vi "login_form.vi"() -> ()   [LabVIEW 2020]
uses:
  <vilib>/httpClient/MultipartData.ctl
  <vilib>/httpClient/LabVIEWHTTPClient.lvlib
panel:
  out "Round tab 2":i32
  in  "Tab Control":enum32{"login", "process"}(tab)
  in  "Cluster":T1
  in  "login":bool
  in  "data":T2[](array[typedef])
  out "Boolean 2":bool
  in  "Boolean":bool
  out "token":string
  out "Hello":string
  in  "stop":bool
  out "date now":string
  out "time":string
  out "body":string
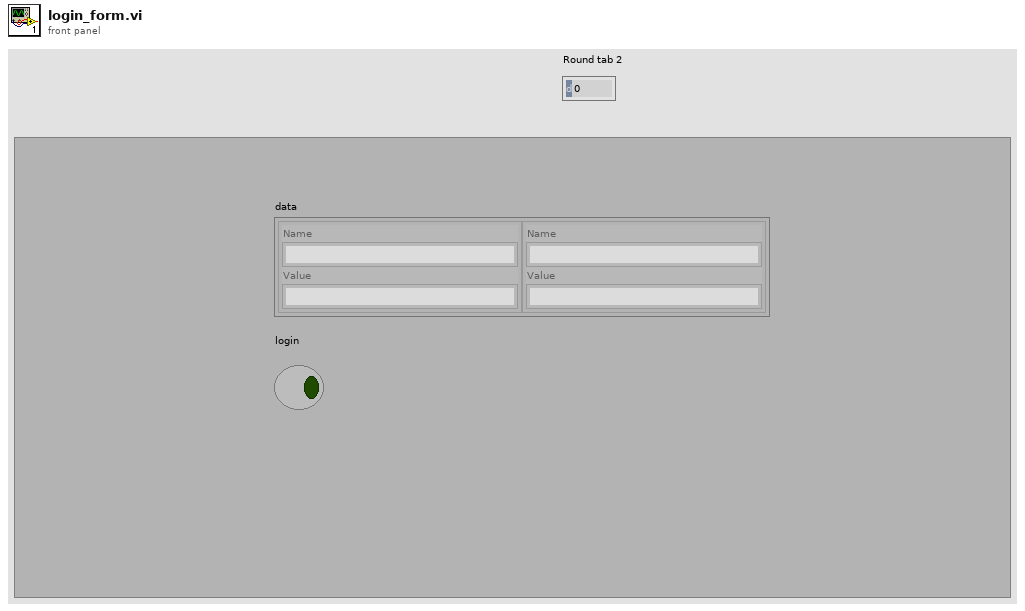
[diagram p1: front panel]
types:
  T1 = cluster{"token":string, "user":cluster{"name":string, "id":string}}
  T2 = typedef "LabVIEWHTTPClient.lvlib/MultipartData.ctl" = cluster{"Name":string, "Value":string, "File":path, "Filename":string, "MIME type":string}
  T3 = typedef "LabVIEWHTTPClient.lvlib/ClientHandle.ctl" = refnum<k1>
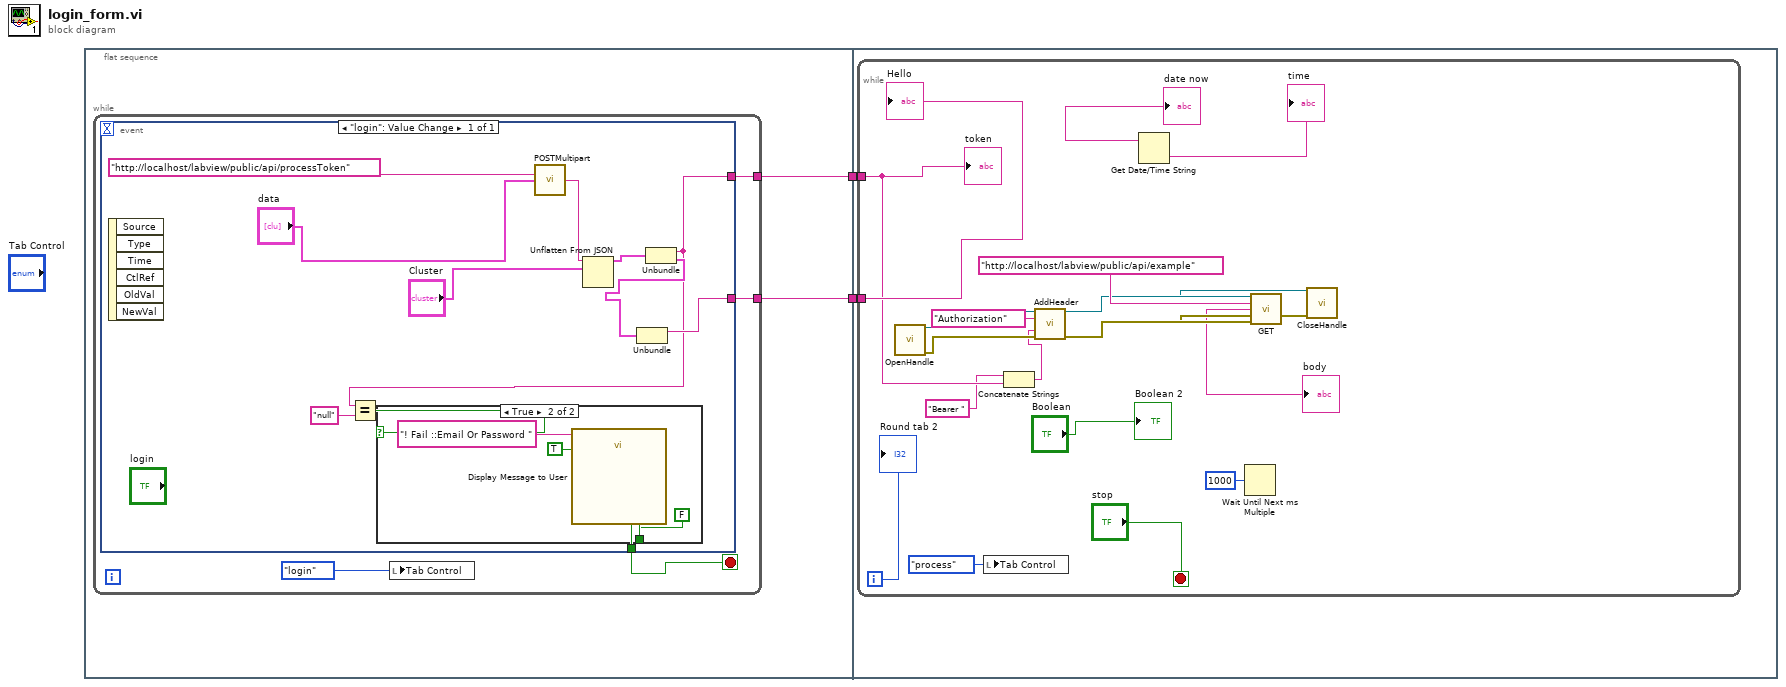
[diagram p0: block diagram]
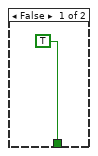
[diagram p2: hidden frame]
diagram:
  n1 = flat-sequence {
    tunnel: [w4] -> w2
    tunnel: [w3] -> w1
    tunnel: w2 -> [w25]
    tunnel: w1 -> [w24]
    frame #0 {
      n2 = while {
        tunnel: [w8] -> w4
        tunnel: [w5] -> w3
        stop <- w7 stop-if-true
        n3 = event shown="[0] \"login\": Value Change" {
          selector: _ -> [_]
          dyn-events: _ -> [_]
          timeout: _ -> [_]
          tunnel: [w13] -> w8
          tunnel: [w12] -> w7
          tunnel: [w9] -> w5
          event "login": Value Change {
            n4 = event-data() -> ()  [unwired: 1 in, 6 out]
            n5 = call <vilib>:"POSTMultipart.vi"("url"="http://localhost/labview/public/api/processToken", "data"="data") -> ("body"=w18:string)  [unwired: 10 in, 3 out]
            n6 = Unflatten From JSON(JSON string=w18, type and defaults="Cluster") -> (value=w15:T1)  [unwired: 5 in, 1 out]
            n7 = Unbundle(w15) -> ("token"=w9:string, "user"=w14:cluster{"name":string, "id":string})
            n8 = Equal?(x=w9, y="null") -> (x = y?=w10:bool)
            n9 = case shown="True" w10 {
              tunnel: [TRUE FALSE] -> w12
              frame False {
              }
              frame True {
                n10 = call "Display Message to User"("Enable"=TRUE, "Message"="! Fail ::Email Or Password ") -> ()  [unwired: 8 in, 2 out]
              }
            }
            n11 = Unbundle(w14) -> ("name"=w13:string)  [unwired: 1 out]
          }
        }
        n12 = local write "Tab Control"(enum32{"login", "process"}."login" ("Tab Control")) -> ()
      }
    }
    frame #1 {
      n13 = while {
        tunnel: w25 -> [w32]
        tunnel: w24 -> [w31]
        i -> [w27]
        stop <- "stop" stop-if-true
        n14 = call <vilib>:"OpenHandle.vi"() -> ("client handle out"=w38:T3, "error out"=w40:errorcluster)  [unwired: 14 in]
        n15 = local write "Tab Control"(enum32{"login", "process"}."process" ("Tab Control")) -> ()
        n16 = Concatenate Strings("Bearer " ("value"), w31) -> (w29:string)
        n17 = call <vilib>:"AddHeader.vi"("client handle"=w38, "header"="Authorization", "value"=w29, "error in (no error)"=w40) -> ("client handle out"=w37:T3, "error out"=w39:errorcluster)  [unwired: 10 in]
        n18 = Get Date/Time String() -> (date string=→"date now":string, time string=→"time":string)  [unwired: 3 in]
        n19 = Wait Until Next ms Multiple(millisecond multiple=u32 1000) -> ()  [unwired: 1 out]
        n20 = call <vilib>:"GET.vi"("client handle"=w37, "url"="http://localhost/labview/public/api/example", "error in (no error)"=w39) -> ("client handle out"=w36:T3, "body"=→"body":string, "error out"=w35:errorcluster)  [unwired: 9 in, 1 out]
        n21 = call <vilib>:"CloseHandle.vi"("client handle"=w36, "error in (no error)"=w35) -> ()  [unwired: 13 in, 1 out]
        "Hello" <- w32
        "token" <- w31
        "Round tab 2" <- w27
        "Boolean 2" <- "Boolean"
      }
    }
  }
